vi "global_vars.vi"() -> ()   [LabVIEW 2023]
panel:
  in  "Stop_button":bool
  in  "Data_value":i32
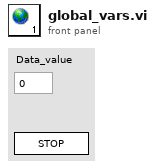
[diagram p1: front panel]
diagram:
